vi "Create.vi"(8 "error in":errorcluster, 11 "IConfiguration":refnum<class "IConfiguration.lvclass">) -> (0 "error out":errorcluster, 3 "IInstrument out":refnum<class "IInstrument.lvclass">)   [LabVIEW 2025, in "Instrument Manager AE.lvlib"]
uses:
  Instrument Manager AE.lvlib
  Interfaces/IInstrument/IInstrument.lvclass
  Interfaces/IConfiguration/IConfiguration.lvclass
  Interfaces/IUnmanaged/IUnmanaged.lvclass
  Interfaces/IConfigure/IConfigure.lvclass
  Interfaces/IConfigurable/IConfigurable.lvclass
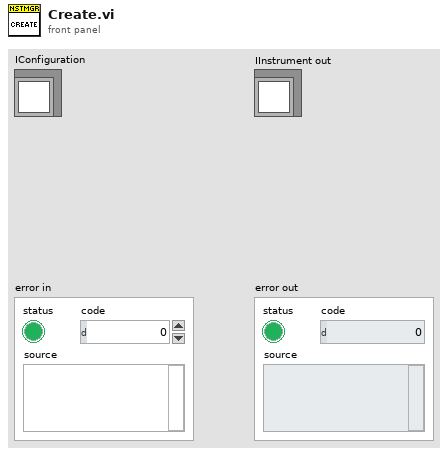
[diagram p1: front panel]
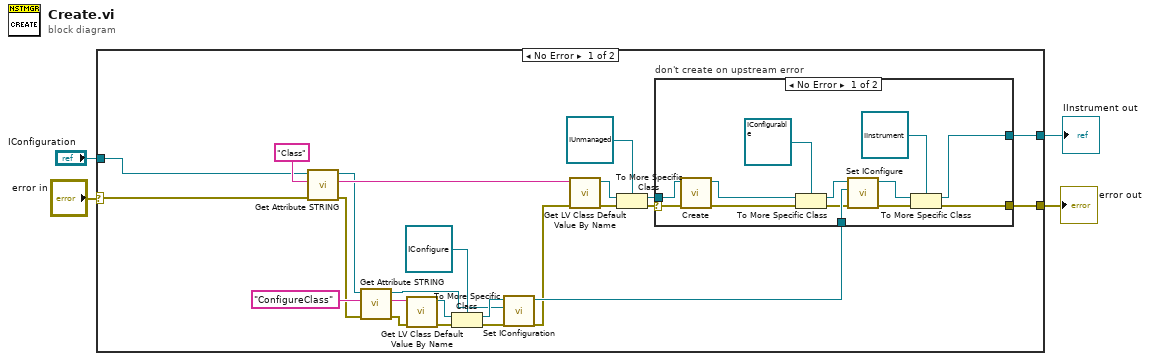
[diagram p0: block diagram]
diagram:
  n1 = case shown="No Error" "error in" {
    selector: "error in" -> [w6 w42]
    tunnel: [w27 w42] -> w3
    tunnel: "IConfiguration" -> [w5 _]
    tunnel: [w26 _] -> w2
    frame No Error {
      n2 = call-dynamic "Get Attribute STRING.vi"("error in"=w6, "Attribute"="Class", "IConfiguration in"=w5) -> ("error out"=w12:errorcluster, "Value"=w24:string, "IConfiguration out"=w14:refnum<class "IConfiguration.lvclass">)  [unwired: 6 in]
      n3 = call-dynamic "Get Attribute STRING.vi"("error in"=w12, "Attribute"="ConfigureClass", "IConfiguration in"=w14) -> ("error out"=w19:errorcluster, "Value"=w20:string, "IConfiguration out"=w9:refnum<class "IConfiguration.lvclass">)  [unwired: 6 in]
      n4 = call <vilib>:"Get LV Class Default Value By Name.vi"("error in (no error)"=w19, "class name"=w20) -> ("error out"=w18:errorcluster, "object"=w17:refnum<class>)  [unwired: 8 in]
      n5 = To More Specific Class(target class=refnum<class "IConfigure.lvclass"> refnum ("IConfigure.lvclass"), reference=w17, error in=w18) -> (specific class reference=w15:refnum<class "IConfigure.lvclass">, error out=w11:errorcluster)
      n6 = call-dynamic "Set IConfiguration.vi"("IConfiguration"=w9, "IConfigure in"=w15) -> ("IConfigure out"=w13:refnum<class "IConfigure.lvclass">)  [unwired: 9 in]
      n7 = call <vilib>:"Get LV Class Default Value By Name.vi"("error in (no error)"=w11, "class name"=w24) -> ("error out"=w22:errorcluster, "object"=w23:refnum<class>)  [unwired: 8 in]
      n8 = To More Specific Class(target class=refnum<class "IUnmanaged.lvclass"> refnum ("IUnmanaged.lvclass"), reference=w23, error in=w22) -> (specific class reference=w7:refnum<class "IUnmanaged.lvclass">, error out=w8:errorcluster)
      n9 = case "don't create on upstream error" shown="No Error" w8 {
        selector: w8 -> [w34 w41]
        tunnel: w13 -> [w39 _]
        tunnel: [w37 w41] -> w27
        tunnel: [w36 _] -> w26
        tunnel: w7 -> [w29 _]
        frame No Error {
          n10 = call-dynamic "Create.vi"("error in"=w34, "IUnmanaged in"=w29) -> ("error out"=w30:errorcluster, "IUnmanaged out"=w28:refnum<class "IUnmanaged.lvclass">)  [unwired: 8 in]
          n11 = To More Specific Class(target class=refnum<class "IConfigurable.lvclass"> refnum ("IConfigurable.lvclass"), reference=w28, error in=w30) -> (specific class reference=w32:refnum<class "IConfigurable.lvclass">, error out=w33:errorcluster)
          n12 = call-dynamic "Set IConfigure.vi"("error in"=w33, "IConfigure"=w39, "IConfigurable in"=w32) -> ("error out"=w35:errorcluster, "IConfigurable out"=w40:refnum<class "IConfigurable.lvclass">)  [unwired: 7 in]
          n13 = To More Specific Class(target class=refnum<class "IInstrument.lvclass"> refnum ("IInstrument.lvclass"), reference=w40, error in=w35) -> (specific class reference=w36:refnum<class "IInstrument.lvclass">, error out=w37:errorcluster)
        }
        frame Error {
        }
      }
    }
    frame Error {
    }
  }
  "error out" <- w3
  "IInstrument out" <- w2
